vi "LaunchEventLogger.vi"(8 "Error In":errorcluster) -> (0 "Error Out":errorcluster, 3 "EventLoggerQueue":refnum<queue>)   [LabVIEW 2019, in "EventLogger.lvlib"]
uses:
  EventLogger.lvlib
  Cluster - MessageCluster.ctl
  Enum - Message.ctl
  EventLogger.vi
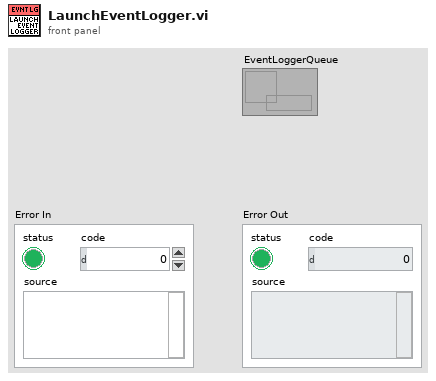
[diagram p1: front panel]
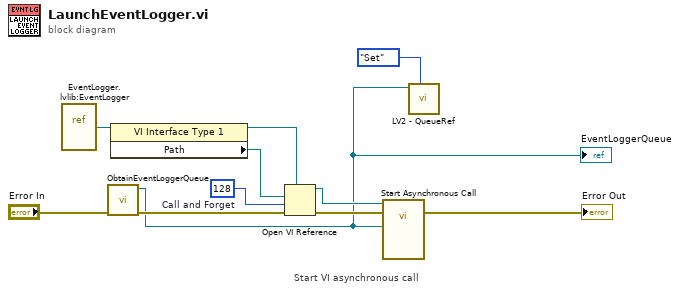
[diagram p0: block diagram]
diagram:
  w6 = 128  # Call and Forget
  # "Start VI asynchronous call"
  n1 = vi-ref "EventLogger.lvlib:EventLogger.vi"() -> (w7:refnum<vi>)
  n2 = call "ObtainEventLoggerQueue.vi"("Error In"="Error In") -> ("Error Out"=w4:errorcluster, "EventLoggerQueue"=w1:refnum<queue>)  [unwired: 9 in]
  "EventLoggerQueue" <- w1
  n3 = property class="VI Interface Type 1"(reference=w7) -> (reference out=w5:refnum<vi>, "Path"=w10:path)  [unwired: 1 in, 1 out]
  n4 = Open VI Reference(type specifier VI Refnum (for type only)=w5, vi path=w10, options=w6, error in (no error)=w4) -> (vi reference=w9:refnum<vi>, error out=w8:errorcluster)  [unwired: 2 in]
  n5 = call-by-ref "Start Asynchronous Call"(reference=w9, error in=w8, "EventLoggerQueue"=w1) -> (error out=→"Error Out":errorcluster)  [unwired: 10 in, 2 out]
  n6 = call "LV2 - QueueRef.vi"("Action"=enum16{"Set", "Get"}."Set", "EventLoggerQueue"=w1) -> ()  [unwired: 9 in, 1 out]
